vi "get Next State.vi"(10 "Playback Controls":T1) -> (3 "Playback State out":T2)   [LabVIEW 2014]
uses:
  Audio/Controls/playback state.ctl
  Controls/Playback Controls.ctl
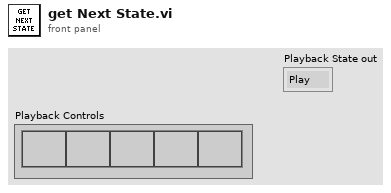
[diagram p1: front panel]
types:
  T1 = typedef "Playback Controls.ctl" = cluster{"Play Button":bool, "Record Button":bool, "Media Stop Button":bool, "Pause Button":bool, "Skip Back Button":bool}
  T2 = typedef "playback state.ctl" = enum16{"Play", "Record", "Stop", "Pause", "Rewind"}
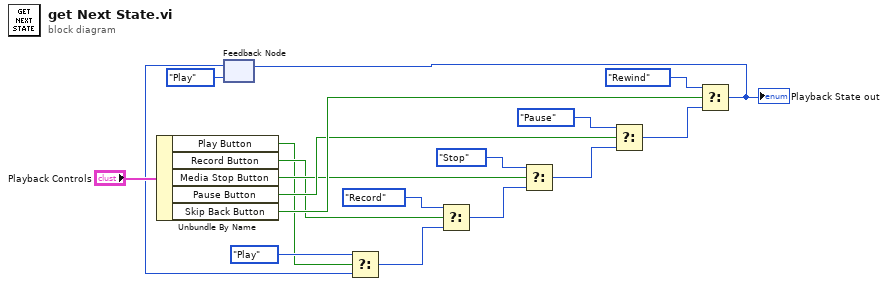
[diagram p0: block diagram]
diagram:
  n1 = Unbundle By Name("Playback Controls") -> ("Play Button"=w5:bool, "Record Button"=w8:bool, "Media Stop Button"=w11:bool, "Pause Button"=w13:bool, "Skip Back Button"=w17:bool)
  n2 = feedback #1(playback_state."Play" ("Playback State")) -> (w2:T2)
  n3 = Select(t=playback_state."Play" ("Playback State"), s=w5, f=w2) -> (s? t:f=w7:T2)
  n4 = Select(t=playback_state."Record", s=w8, f=w7) -> (s? t:f=w10:T2)
  n5 = Select(t=playback_state."Stop", s=w11, f=w10) -> (s? t:f=w14:T2)
  n6 = Select(t=playback_state."Pause", s=w13, f=w14) -> (s? t:f=w16:T2)
  n7 = Select(t=playback_state."Rewind", s=w17, f=w16) -> (s? t:f=w3:T2)
  "Playback State out" <- w3
  n8 = feedback-in #1(w3) -> ()
